vi "Init Waveforms.vi"(8 "error in (no error)":errorcluster, 11 "Async Input in":T4={"Device Ref"=18446744073709551615, "Waveforms"=[], "Channels"={"Command Chan Refs"=[], "Command Data Refs"=[], "Command Values"=[], "Status Chan Refs"=[], "Status Data Refs"=[], "Status Values"=[], "System Time"={"System Time"=timestamp(0 s since 1904-01-01), "Data Reference"=0, "Absolute Time Channel Data Ref"=0, "Get Date-Time Channel Data Ref"=0}, "Trigger Chan Refs"=[], "Trigger Data Refs"=[], "Trigger Values"=[]}, "Waveform Logs"=[], "Communication"={"Async Status"=refnum, "Wfm Comm Properties"={"WPL"={"Custom Queue Size"=1, "Use Custom Queue Size?"=FALSE}}, "Shutdown Event"=refnum, "Trigger Event"=refnum, "New File Event"=refnum, "Log Queues"=[], "Async VI Ref"=refnum}, "error"={"status"=FALSE, "code"=0, "source"=""}} {"Device Ref" format="%.0x"; "Channels"."Trigger Data Refs"."Data Reference" format="%.0x"; "Channels"."Trigger Chan Refs" format="%.0x"; "Channels"."System Time"."Get Date-Time Channel Data Ref" format="%.0x"; "Channels"."System Time"."Absolute Time Channel Data Ref" format="%.0x"; "Channels"."System Time"."Channel Data Reference" format="%.0x"; "Channels"."Status Data Refs"."Data Reference" format="%.0x"; "Channels"."Command Data Refs"."Data Reference" format="%.0x"; "Channels"."Status Chan Refs" format="%.0x"; "Channels"."Command Chan Refs" format="%.0x"; "Waveforms"."Waveform Ref in" format="%.0x"; "Waveform Logs"."Node ID" format="%.0x"; "Waveform Logs"."TDMS Error Code"."Data Ref" format="%.0x"; "Waveform Logs"."Missed Samples"."Data Ref" format="%.0x"; "Waveform Logs"."File Status"."Data Ref" format="%.0x"; "Waveform Logs"."Start New File"."Data Ref" format="%.0x"; "Waveform Logs"."Logging Enabled"."Data Ref" format="%.0x"; "Waveform Logs"."Stop Trigger"."Node Data Ref" format="%.0x"; "Waveform Logs"."Stop Trigger"."Node ID" format="%.0x"; "Waveform Logs"."Start Trigger"."Node Data Ref" format="%.0x"; "Waveform Logs"."Start Trigger"."Node ID" format="%.0x"}) -> (0 "error out":errorcluster, 1 "Wfm Buffers":refnum<data-value>[](array[refnum]), 2 "Async Data out":T1, 3 "Async Input out":T4={"Device Ref"=18446744073709551615, "Waveforms"=[], "Channels"={"Command Chan Refs"=[], "Command Data Refs"=[], "Command Values"=[], "Status Chan Refs"=[], "Status Data Refs"=[], "Status Values"=[], "System Time"={"System Time"=timestamp(0 s since 1904-01-01), "Data Reference"=0, "Absolute Time Channel Data Ref"=0, "Get Date-Time Channel Data Ref"=0}, "Trigger Chan Refs"=[], "Trigger Data Refs"=[], "Trigger Values"=[]}, "Waveform Logs"=[], "Communication"={"Async Status"=refnum, "Wfm Comm Properties"={"WPL"={"Custom Queue Size"=1, "Use Custom Queue Size?"=FALSE}}, "Shutdown Event"=refnum, "Trigger Event"=refnum, "New File Event"=refnum, "Log Queues"=[], "Async VI Ref"=refnum}, "error"={"status"=FALSE, "code"=0, "source"=""}} {"Device Ref" format="%.0x"; "Channels"."Trigger Data Refs"."Data Reference" format="%.0x"; "Channels"."Trigger Chan Refs" format="%.0x"; "Channels"."System Time"."Get Date-Time Channel Data Ref" format="%.0x"; "Channels"."System Time"."Absolute Time Channel Data Ref" format="%.0x"; "Channels"."System Time"."Channel Data Reference" format="%.0x"; "Channels"."Status Data Refs"."Data Reference" format="%.0x"; "Channels"."Command Data Refs"."Data Reference" format="%.0x"; "Channels"."Status Chan Refs" format="%.0x"; "Channels"."Command Chan Refs" format="%.0x"; "Waveforms"."Waveform Ref in" format="%.0x"; "Waveform Logs"."Node ID" format="%.0x"; "Waveform Logs"."TDMS Error Code"."Data Ref" format="%.0x"; "Waveform Logs"."Missed Samples"."Data Ref" format="%.0x"; "Waveform Logs"."File Status"."Data Ref" format="%.0x"; "Waveform Logs"."Start New File"."Data Ref" format="%.0x"; "Waveform Logs"."Logging Enabled"."Data Ref" format="%.0x"; "Waveform Logs"."Stop Trigger"."Node Data Ref" format="%.0x"; "Waveform Logs"."Stop Trigger"."Node ID" format="%.0x"; "Waveform Logs"."Start Trigger"."Node Data Ref" format="%.0x"; "Waveform Logs"."Start Trigger"."Node ID" format="%.0x"})   [LabVIEW 2012, in "Waveform Data Logger Engine.lvlib"]
uses:
  Waveform Data Logger Engine.lvlib
  Types/RT Data.ctl
  <vilib>/NI Veristand/Custom Device API/Custom Device Item Ref.ctl
  Types/Inline Waveform Info.ctl
  <vilib>/NI Veristand/Custom Device API/Waveform Data Reference.ctl
  Classes/Waveforms/Waveform Receive/Associated Log.ctl
  <vilib>/NI Veristand/Custom Device API/Custom Device Waveform DataType.ctl
  Types/Channels.ctl
  <vilib>/NI Veristand/Custom Device API/Block Data Reference.ctl
  <vilib>/NI Veristand/Custom Device API/Data Reference.ctl
  Types/System Time.ctl
  Types/Inline Waveform Log Info.ctl
  Shared/Classes/Log File Specifications/Waveform TDMS Log File Specification/Waveform TDMS Log File Specification.lvclass
  Classes/Triggers/Trigger/Trigger.lvclass
  Types/Inline Log Waveform.ctl
  Types/Trigger Settings.ctl
  Types/Log Status.ctl
  Types/Channel.ctl
  Types/Communication.ctl
  Types/Async Status.ctl
  Types/Async State.ctl
  <vilib>/NI Veristand/Custom Device Waveform API/Communication Properties.ctl
  Types/Trigger Event Data.ctl
  Types/Trigger Received.ctl
  Types/New File Event Data.ctl
  Types/Log Queues.ctl
  Types/Async Data.ctl
  <vilib>/NI Veristand/Custom Device Waveform API/Multiple Waveforms Read (DBL)/Multiple Waveforms Read (DBL).lvclass
  Classes/Waveforms/Utilities/Reference Dictionary/Reference Dictionary.lvclass
  Types/Wfm Acq Data.ctl
  Classes/Waveforms/Waveform Receive/Waveform Receive.lvclass
  Classes/Waveforms/Waveform Log/Waveform Log.lvclass
  Types/Async Communication.ctl
  Types/Check File Loop Cmd.ctl
  Classes/Waveforms/Buffer/Waveform Buffer/Waveform Buffer.lvclass
  Classes/Waveforms/Buffer/Waveform Buffer/Buffer Data Type.ctl
  <vilib>/NI Veristand/Custom Device Waveform API/Multiple Waveforms Read (DBL)/NI VeriStand - Open Multiple Waveforms Read Session (DBL).vi
  <vilib>/NI VeriStand/Custom Device Waveform API/NI_VS Custom Device Waveform API.lvlib
  <vilib>/NI VeriStand/Custom Device API/Custom Device API.lvlib
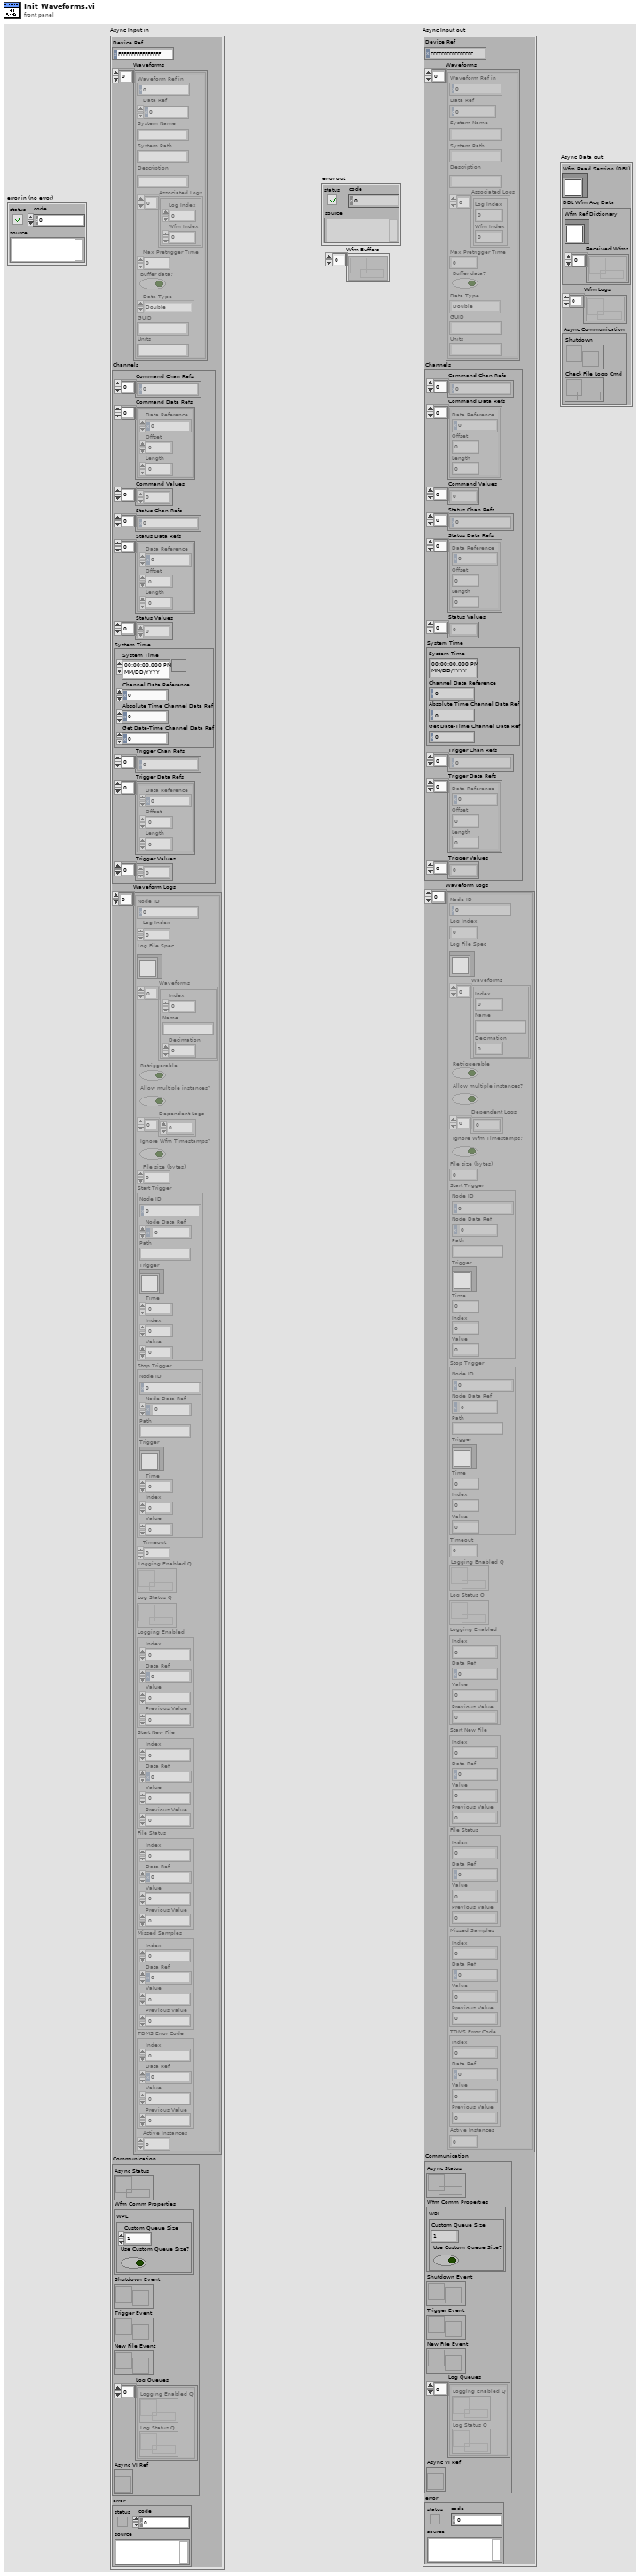
[diagram p1: front panel]
types:
  T1 = typedef "Waveform Data Logger Engine.lvlib/Async Data.ctl" = cluster{"Wfm Read Session (DBL)":refnum<class "Multiple Waveforms Read (DBL).lvclass">, "DBL Wfm Acq Data":T2, "Wfm Logs":refnum<data-value>[], "Async Communication":T3}
  T2 = typedef "Waveform Data Logger Engine.lvlib/Wfm Acq Data.ctl" = cluster{"Wfm Ref Dictionary":refnum<class "Reference Dictionary.lvclass">, "Received Wfms":refnum<data-value>[]}
  T3 = typedef "Waveform Data Logger Engine.lvlib/Async Communication.ctl" = cluster{"Shutdown":refnum<user-event>, "Check File Loop Cmd":refnum<queue>}
  T4 = typedef "Waveform Data Logger Engine.lvlib/RT Data.ctl" = cluster{"Device Ref":T5, "Waveforms":T6[], "Channels":T10, "Waveform Logs":T14[], "Communication":T18, "error":errorcluster}
  T5 = typedef "Custom Device API.lvlib/Custom Device Item Ref.ctl" = u64
  T6 = typedef "Waveform Data Logger Engine.lvlib/Inline Waveform Info.ctl" = cluster{"Waveform Ref in":T5, "Data Ref":T7, "System Name":string, "System Path":string, "Description":string, "Associated Logs":T8[], "Max Pretrigger Time":dbl, "Buffer data?":bool, "Data Type":T9, "GUID":string, "Units":string}
  T7 = typedef "Custom Device API.lvlib/Waveform Data Reference.ctl" = i32
  T8 = typedef "Waveform Data Logger Engine.lvlib/Waveform Receive.lvclass/Associated Log.ctl" = cluster{"Log Index":i32, "Wfm Index":i32}
  T9 = typedef "Custom Device API.lvlib/Custom Device Waveform DataType.ctl" = enum16{"Double", "Complex Double"}
  T10 = typedef "Waveform Data Logger Engine.lvlib/Channels.ctl" = cluster{"Command Chan Refs":T5[], "Command Data Refs":T11[], "Command Values":dbl[], "Status Chan Refs":T5[], "Status Data Refs":T11[], "Status Values":dbl[], "System Time":T13, "Trigger Chan Refs":T5[], "Trigger Data Refs":T11[], "Trigger Values":dbl[]}
  T11 = typedef "Custom Device API.lvlib/Block Data Reference.ctl" = cluster{"Data Reference":T12, "Offset":i32, "Length":i32}
  T12 = typedef "Custom Device API.lvlib/Data Reference.ctl" = i32
  T13 = typedef "Waveform Data Logger Engine.lvlib/System Time.ctl" = cluster{"System Time":timestamp, "Data Reference":T12, "Absolute Time Channel Data Ref":T12, "Get Date-Time Channel Data Ref":T12}
  T14 = typedef "Waveform Data Logger Engine.lvlib/Inline Waveform Log Info.ctl" = cluster{"Node ID":T5, "Log Index":i32, "Log File Spec":refnum<class "Waveform TDMS Log File Specification.lvclass">, "Waveforms":T15[], "Retriggerable":bool, "Allow multiple instances?":bool, "Dependent Logs":i32[], "Ignore Wfm Timestamps?":bool, "File size (bytes)":i64, "Start Trigger":T16, "Stop Trigger":T16, "Timeout":dbl, "Logging Enabled Q":refnum<queue>, "Log Status Q":refnum<queue>, "Logging Enabled":T17, "Start New File":T17, "File Status":T17, "Missed Samples":T17, "TDMS Error Code":T17, "Active Instances":i32}
  T15 = typedef "Waveform Data Logger Engine.lvlib/Inline Log Waveform.ctl" = cluster{"Index":i32, "Name":string, "Decimation":u32}
  T16 = typedef "Waveform Data Logger Engine.lvlib/Trigger Settings.ctl" = cluster{"Node ID":T5, "Node Data Ref":i32, "Path":string, "Trigger":refnum<class "Trigger.lvclass">, "Time":dbl, "Index":i32, "Value":dbl}
  T17 = typedef "Waveform Data Logger Engine.lvlib/Channel.ctl" = cluster{"Index":i32, "Data Ref":T12, "Value":dbl, "Previous Value":dbl}
  T18 = typedef "Waveform Data Logger Engine.lvlib/Communication.ctl" = cluster{"Async Status":refnum<queue>, "Wfm Comm Properties":T19, "Shutdown Event":refnum<user-event>, "Trigger Event":refnum<user-event>, "New File Event":refnum<user-event>, "Log Queues":T20[], "Async VI Ref":refnum<vi>}
  T19 = typedef "NI_VS Custom Device Waveform API.lvlib/Communication Properties.ctl" = cluster{"WPL":cluster{"Custom Queue Size":i32, "Use Custom Queue Size?":bool}}
  T20 = typedef "Waveform Data Logger Engine.lvlib/Log Queues.ctl" = cluster{"Logging Enabled Q":refnum<queue>, "Log Status Q":refnum<queue>}
  T21 = typedef "Waveform Data Logger Engine.lvlib/Waveform Buffer.lvclass/Buffer Data Type.ctl" = enum16{"Double", "ComplexDouble"}
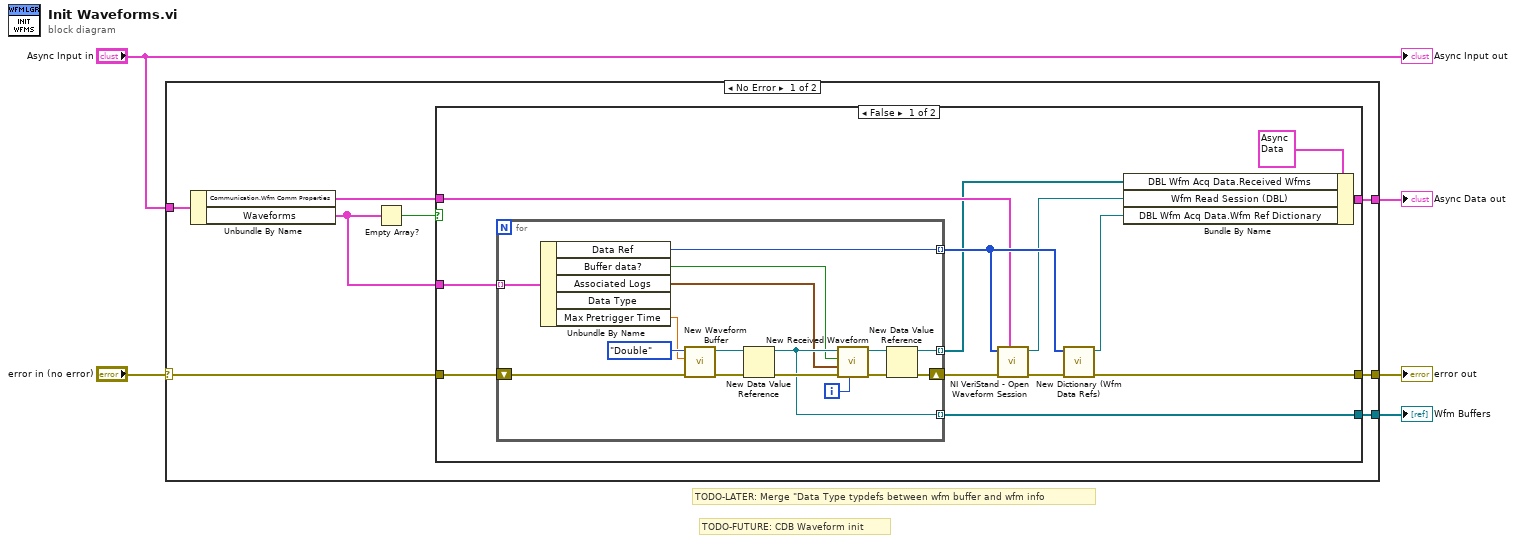
[diagram p0: block diagram]
diagram:
  # "TODO-FUTURE: CDB Waveform init"
  # "TODO-LATER: Merge \"Data Type typdefs between wfm buffer and wfm info"
  n1 = case shown="No Error" "error in (no error)" {
    selector: "error in (no error)" -> [w9 w44]
    tunnel: [w13 w44] -> w4
    tunnel: [w12 _] -> w3
    tunnel: "Async Input in" -> [w10 _]
    tunnel: [w8 _] -> w2
    frame No Error {
      n2 = Unbundle By Name(w10) -> ("Communication.Wfm Comm Properties"=w11:T19, "Waveforms"=w7:T6[])
      n3 = Empty Array?(array=w7) -> (empty?=w6:bool)
      n4 = case shown="False" w6 {
        tunnel: [w24 w43] -> w13
        tunnel: [w21 _] -> w12
        tunnel: w11 -> [w20 _]
        tunnel: w9 -> [w19 w43]
        tunnel: [w18 _] -> w8
        tunnel: w7 -> [w14 _]
        frame False {
          n5 = for {
            tunnel: w14 -> [w42] mode=indexing
            tunnel: [w41] -> w26 mode=indexing
            shift-right: [w35] -> w17
            shift-left: w19 -> [w39]
            tunnel: [w29] -> w18 mode=indexing
            tunnel: [w32] -> w16 mode=indexing
            i -> [w30]
            n6 = Unbundle By Name(w42) -> ("Data Ref"=w41:T7, "Buffer data?"=w28:bool, "Associated Logs"=w27:T8[], "Max Pretrigger Time"=w31:dbl)  [unwired: 1 out]
            n7 = call "New Waveform Buffer.vi"("error in (no error)"=w39, "Buffer Duration"=w31, "Buffer Data Type"=Buffer_Data_Type."Double") -> ("error out"=w38:errorcluster, "Waveform Buffer out"=w37:refnum<class "Waveform Buffer.lvclass">)  [unwired: 7 in]
            n8 = New Data Value Reference(data value=w37, error in=w38) -> (data value reference=w29:refnum<data-value>, error out=w36:errorcluster)
            n9 = call "New Received Waveform.vi"("Wfm Index"=w30, "error in (no error)"=w36, "Associated Logs"=w27, "Buffer data?"=w28, "Wfm Buffer Ref"=w29) -> ("error out"=w34:errorcluster, "Waveform Receive out"=w33:refnum<class "Waveform Receive.lvclass">)  [unwired: 5 in]
            n10 = New Data Value Reference(data value=w33, error in=w34) -> (data value reference=w32:refnum<data-value>, error out=w35:errorcluster)
          }
          n11 = call-poly <vilib>:"NI VeriStand - Open Waveform Session.vi"("Communication Properties"=w20, "error in (no error)"=w17, "DBL Waveform Data References"=w26) -> ("error out"=w25:errorcluster, "Multiple Waveforms Read Session (DBL)"=w23:refnum<class "Multiple Waveforms Read (DBL).lvclass">)  [unwired: 7 in]
          n12 = call "New Dictionary (Wfm Data Refs).vi"("error in (no error)"=w25, "Wfm Data Refs"=w26) -> ("error out"=w24:errorcluster, "Dictionary out"=w22:refnum<class "Reference Dictionary.lvclass">)  [unwired: 8 in]
          n13 = Bundle By Name(cluster=T1 {"Wfm Read Session (DBL)"=refnum, "DBL Wfm Acq Data"={"Wfm Ref Dictionary"=refnum, "Received Wfms"=[]}, "Wfm Logs"=[], "Async Communication"={"Shutdown"=refnum, "Check File Loop Cmd"=refnum}} ("Async Data"), "DBL Wfm Acq Data.Received Wfms"=w16, "Wfm Read Session (DBL)"=w23, "DBL Wfm Acq Data.Wfm Ref Dictionary"=w22) -> (w21:T1)
        }
        frame True {
        }
      }
    }
    frame Error {
    }
  }
  "Async Data out" <- w3
  "error out" <- w4
  "Wfm Buffers" <- w2
  "Async Input out" <- "Async Input in"
